vi "Report_Type.vi"(8 "error in (no error)":errorcluster, 11 "IB_DotNET in":refnum<class "IB_DotNET.lvclass">) -> (0 "error out":errorcluster, 2 "type":string, 3 "IB_DotNET out":refnum<class "IB_DotNET.lvclass">)   [LabVIEW 2020, in "IB_DotNET.lvclass"]
uses:
  <vilib>/AppBuilder/IB_Classes/Source/Container/Build/NET/IB_DotNET.lvclass
  <vilib>/AppBuilder/IB_Classes/Source/Container/Build/NET/IB_DotNET.lvclass/IB_DotNET.ctl
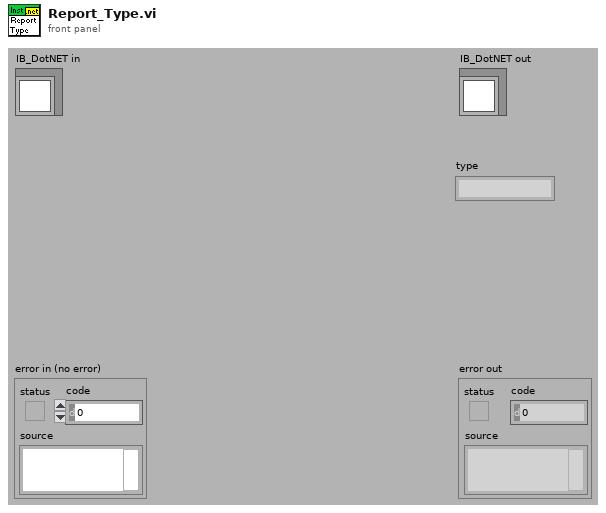
[diagram p1: front panel]
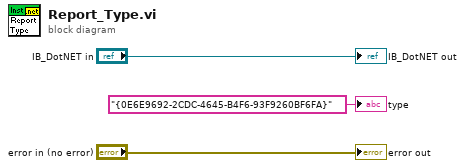
[diagram p0: block diagram]
diagram:
  "error out" <- "error in (no error)"
  "IB_DotNET out" <- "IB_DotNET in"
  "type" <- "{0E6E9692-2CDC-4645-B4F6-93F9260BF6FA}" ("type")
